vi "DAQmx Start Trigger (Analog Edge).vi"(0 "task/channels in":refnum<k21>, 5 "source":string, 7 "slope":i32(ring)=10280 items=["Rising"=10280, "Falling"=10171], 9 "level":dbl format="%0.2f", 11 "error in":errorcluster) -> (4 "task out":refnum<k21>, 15 "error out":errorcluster)   [LabVIEW 2011]
doc: "Configures the task to start acquiring or generating samples when an analog signal crosses the level you specify."
uses:
  C:/Program Files/National Instruments/LabVIEW 2011/resource/objmgr/daqmx.rc
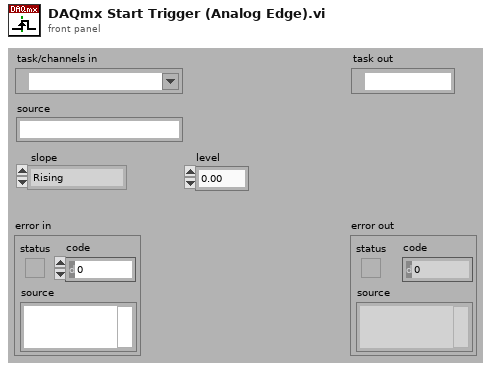
[diagram p1: front panel]
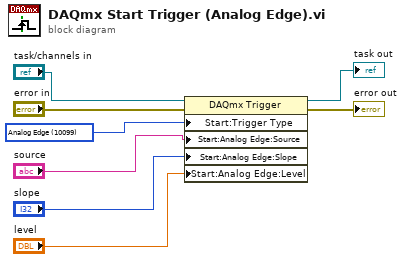
[diagram p0: block diagram]
diagram:
  w3 = 10099 items=["Analog Edge"=10099, "Digital Edge"=10150, "Analog Window"=10103, "None"=10230] ("Start:Trigger Type")
  n1 = property class="DAQmx Trigger"(reference="task/channels in", error in="error in", "Start:Trigger Type"=w3, "Start:Analog Edge:Source"="source", "Start:Analog Edge:Slope"="slope", "Start:Analog Edge:Level"="level") -> (reference out=→"task out":refnum<k21>, error out=→"error out":errorcluster)
